vi "Open Connection.vi"(6 "timeout":i32=-1, 8 "error in (no error)":errorcluster, 9 "remote port":u16=54165, 10 "IP":string="200.131.64.48", 11 "TCPIP in":refnum<class "TCPIP.lvclass">) -> (0 "error out":errorcluster, 3 "TCPIP out":refnum<class "TCPIP.lvclass">)   [LabVIEW 2018, in "TCPIP.lvclass"]
uses:
  TCPIP.lvclass
  TCPIP.lvclass/TCPIP.ctl
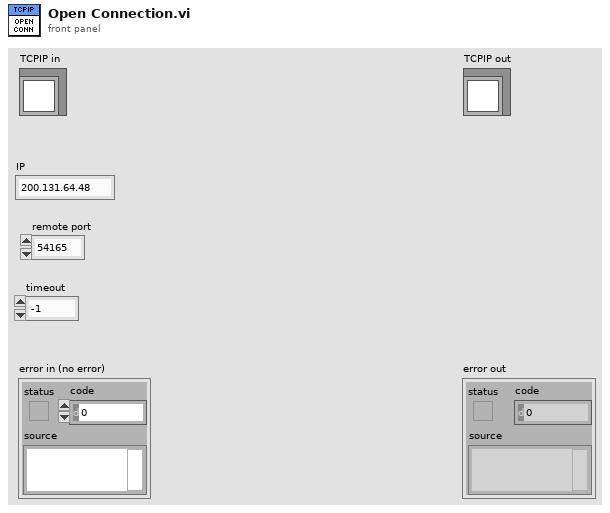
[diagram p1: front panel]
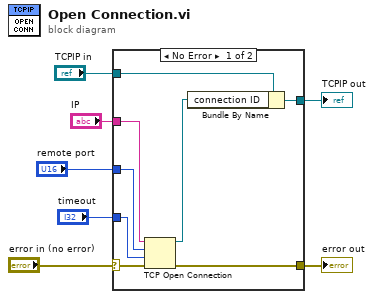
[diagram p0: block diagram]
diagram:
  n1 = case shown="No Error" "error in (no error)" {
    selector: "error in (no error)" -> [w12 w17]
    tunnel: [w11 w17] -> w6
    tunnel: [w14 w16] -> w4
    tunnel: "TCPIP in" -> [w15 w16]
    tunnel: "IP" -> [w10 _]
    tunnel: "remote port" -> [w9 _]
    tunnel: "timeout" -> [w8 _]
    frame No Error {
      n2 = TCP Open Connection(address=w10, remote port or service name=w9, timeout ms (60000)=w8, error in (no error)=w12) -> (connection ID=w13:refnum<k5>, error out=w11:errorcluster)  [unwired: 1 in]
      n3 = Bundle By Name(cluster=w15, "connection ID"=w13) -> (w14:refnum<class "TCPIP.lvclass">)
    }
    frame Error {
    }
  }
  "error out" <- w6
  "TCPIP out" <- w4
